vi "Shoot Feeder.vi"(2 "Enum":T5(ring)) -> ()   [LabVIEW 2011]
uses:
  TypeDefs/PWM Module 1.ctl
  <vilib>/Rock Robotics/SystemInterfaces/Typedef/FPGA_TypedefDigitalModule.ctl
  <vilib>/Rock Robotics/SystemInterfaces/DIO/FPGA_DIOPWMChannel.ctl
  <vilib>/Rock Robotics/SystemInterfaces/DIO/FPGA_DIORelayChannel.ctl
  <vilib>/Rock Robotics/WPI/MotorControl/WPI_MotorControlOpen Victor.vi
panel:
  in  "PWM Module (DIO A)":T1={"Module"=enum."Digital Module 1", "Shooter Wheel"=enum."PWM 1", "Unassigned"=enum."PWM 2", "Unassigned"=enum."PWM 3", "Unassigned"=enum."PWM 4", "Unassigned"=enum."PWM 5", "Arm Servo"=enum."PWM 6", "Arm"=enum."PWM 7", "Ball Intake"=enum."PWM 8", "Conveyor Belt"=enum."PWM 9", "Shooter Feeder"=enum."PWM 10", "Camera Light"=enum."Relay 1", "Unassigned"=enum."Relay 2", "Unassigned"=enum."Relay 3", "Unassigned"=enum."Relay 4", "Unassigned"=enum."Relay 5", "Unassigned"=enum."Relay 6", "Unassigned"=enum."Relay 7", "Unassigned "=enum."Relay 8"}
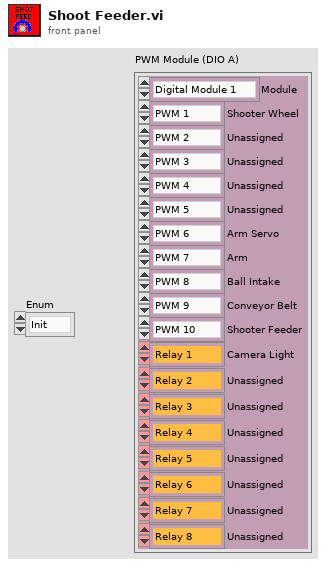
[diagram p1: front panel]
types:
  T1 = typedef "PWM Module 1.ctl" = cluster{"Module":T2, "Shooter Wheel":T3, "Unassigned":T3, "Unassigned":T3, "Unassigned":T3, "Unassigned":T3, "Arm Servo":T3, "Arm":T3, "Ball Intake":T3, "Conveyor Belt":T3, "Shooter Feeder":T3, "Camera Light":T4, "Unassigned":T4, "Unassigned":T4, "Unassigned":T4, "Unassigned":T4, "Unassigned":T4, "Unassigned":T4, "Unassigned ":T4}
  T2 = typedef "FPGA_TypedefDigitalModule.ctl" = enum16{"Digital Module 1", "Digital Module 2"}
  T3 = typedef "FPGA_DIOPWMChannel.ctl" = enum8{"PWM 1", "PWM 2", "PWM 3", "PWM 4", "PWM 5", "PWM 6", "PWM 7", "PWM 8", "PWM 9", "PWM 10", "Invalid"}
  T4 = typedef "FPGA_DIORelayChannel.ctl" = enum8{"Relay 1", "Relay 2", "Relay 3", "Relay 4", "Relay 5", "Relay 6", "Relay 7", "Relay 8", "Invalid"}
  T5 = enum16{"Init", "Stop", "Shoot", "Reverse", "End"}
  T6 = typedef "WPI_MotorControlDeviceRef.ctl" = cluster{"DeviceStatus":errorcluster, "Type":enum16{"PWM", "CAN"}, "PWM":cluster{"Digital Module":T2, "PWM Channel":T3, "DeadBand":T7}, "CAN":cluster{"Device Number":u8, "Control Mode":T8, "Semaphore":T9, "Max Vout":dbl}, "Invert":bool, "TransformRef":T10, "InvTransformRef":T10}
  T7 = typedef "WPI_PWMDeadband.ctl" = cluster{"Name":string, "maxPositivePwm":i32, "minPositivePwm":i32, "centerPwm":i32, "maxNegativePwm":i32, "minNegativePwm":i32, "angularRange":u16}
  T8 = typedef "WPI_CANJaguar_ControlMode.ctl" = enum8{"Percent VBus", "Current", "Speed", "Position", "Voltage"}
  T9 = typedef "Semaphore RefNum" = refnum<k1>
  T10 = typedef "WPI_PWMTransform_ConPane.ctl" = refnum<vi>
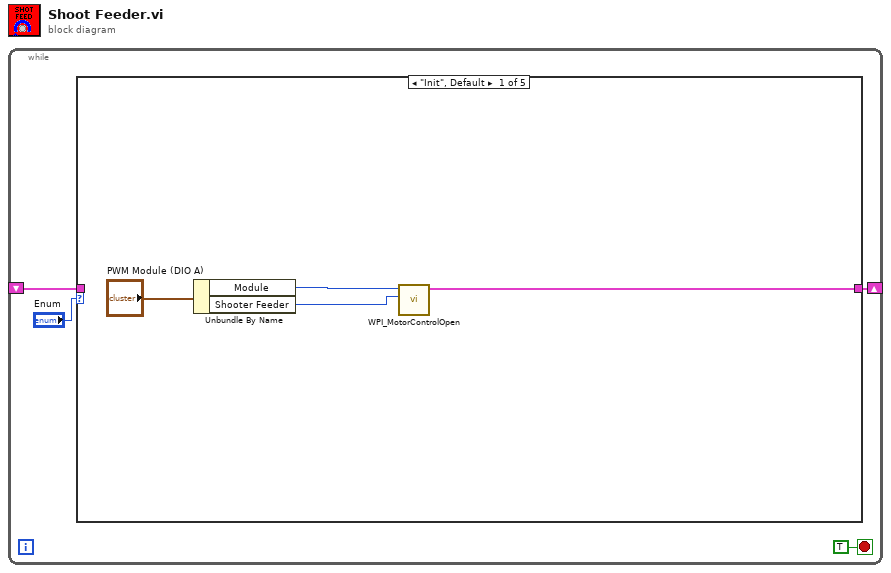
[diagram p0: block diagram]
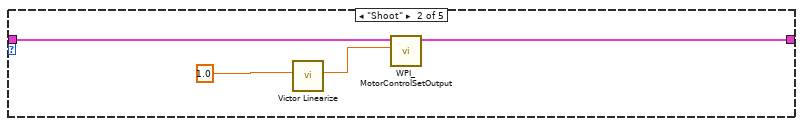
[diagram p2: hidden frame]
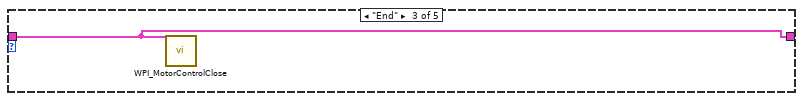
[diagram p3: hidden frame]
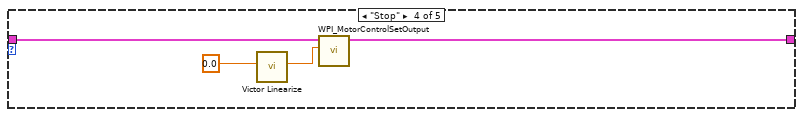
[diagram p4: hidden frame]
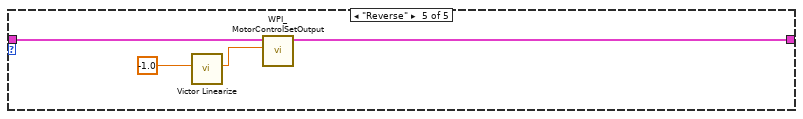
[diagram p5: hidden frame]
diagram:
  n1 = while {
    shift-right: [w3] -> _
    shift-left: _ -> [w2]
    stop <- TRUE stop-if-true
    n2 = case shown="\"Init\", Default" "Enum" {
      tunnel: [w5 w11 w13 w16 w20] -> w3
      tunnel: w2 -> [_ w12 w13 w17 w21]
      frame "Init", Default {
        n3 = Unbundle By Name("PWM Module (DIO A)") -> ("Module"=w7:T2, "Shooter Feeder"=w6:T3)
        n4 = call-poly <vilib>:"WPI_MotorControlOpen.vi"("PWM Channel"=w6, "Digital Module (Module 1)"=w7) -> ("MotorControlDeviceRef"=w5:T6)  [unwired: 8 in, 1 out]
      }
      frame "Shoot" {
        n5 = call "Victor Linearize.vi"("Goal Speed"=1.0 ("Output")) -> ("Output"=w9:dbl)  [unwired: 10 in]
        n6 = call <vilib>:"WPI_MotorControlSetOutput.vi"("Output"=w9, "MotorControlDevRef"=w12) -> ("MotorControlDevRef"=w11:T6)  [unwired: 8 in, 1 out]
      }
      frame "End" {
        n7 = call <vilib>:"WPI_MotorControlClose.vi"("MotorControlDevRef"=w13) -> ()  [unwired: 10 in, 1 out]
      }
      frame "Stop" {
        n8 = call "Victor Linearize.vi"("Goal Speed"=0.0 ("Output")) -> ("Output"=w14:dbl)  [unwired: 10 in]
        n9 = call <vilib>:"WPI_MotorControlSetOutput.vi"("Output"=w14, "MotorControlDevRef"=w17) -> ("MotorControlDevRef"=w16:T6)  [unwired: 8 in, 1 out]
      }
      frame "Reverse" {
        n10 = call "Victor Linearize.vi"("Goal Speed"=-1.0 ("Output")) -> ("Output"=w18:dbl)  [unwired: 10 in]
        n11 = call <vilib>:"WPI_MotorControlSetOutput.vi"("Output"=w18, "MotorControlDevRef"=w21) -> ("MotorControlDevRef"=w20:T6)  [unwired: 8 in, 1 out]
      }
    }
  }
